vi "stc31-csv-to-data.vi"(10 "sensor-name":string, 11 "sensor-csv-input":string) -> (1 "STC31: Temp (degC)":dbl format="%.2f", 2 "STC31: CO2 (ppm)":dbl format="%.2f", 3 "STC31: data output":T1 {"CO2 (ppm)" format="%.2f"})   [LabVIEW 2021]
uses:
  STC31.ctl
  <vilib>/regexp/Match Regular Expression.xnode
panel:
  out "STC31: Temp":string
  out "STC31: CO2":string
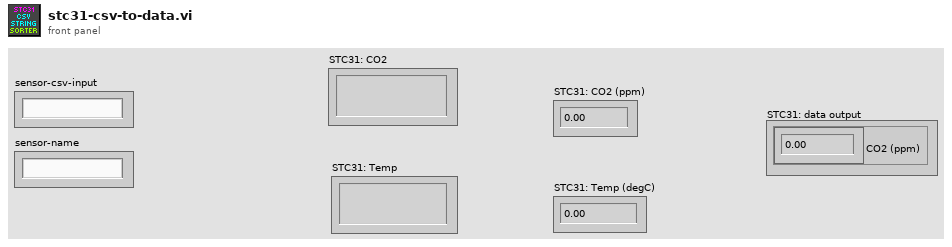
[diagram p1: front panel]
types:
  T1 = typedef "STC31.ctl" = cluster{"CO2 (ppm)":dbl}
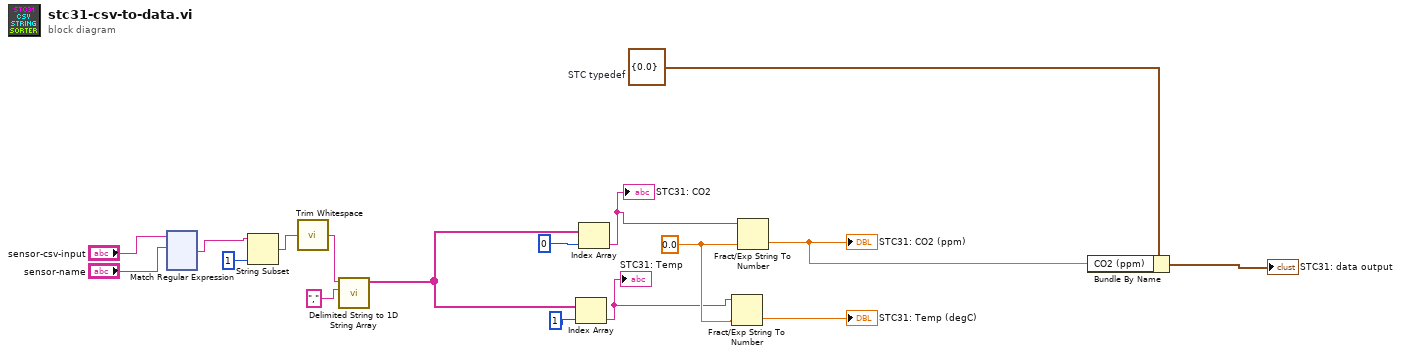
[diagram p0: block diagram]
diagram:
  w15 = T1 {"CO2 (ppm)"=0.0}  # STC typedef
  w17 = 0.0
  n1 = xnode "Match Regular Expression"("input string"="sensor-csv-input", "regular expression"="sensor-name") -> ("after match"=w1:string)  [unwired: 4 in, 4 out]
  n2 = String Subset(string=w1, offset (0)=1) -> (substring=w2:string)  [unwired: 1 in]
  n3 = call <vilib>:"Trim Whitespace.vi"("string"=w2) -> ("trimmed string"=w12:string)  [unwired: 1 in]
  n4 = call <vilib>:"Delimited String to 1D String Array.vi"("delimiter"=",", "delimited string"=w12) -> ("string array"=w6:string[])  [unwired: 9 in]
  n5 = Index Array(array=w6, index=1 ("y")) -> (element=w4:string)
  "STC31: Temp" <- w4
  n6 = Index Array "Index Array"(array=w6, index=0) -> (element=w5:string)
  "STC31: CO2" <- w5
  n7 = Fract/Exp String To Number(string=w4, default (0 dbl)=w17) -> (number=→"STC31: Temp (degC)":dbl)  [unwired: 2 in, 1 out]
  n8 = Fract/Exp String To Number(string=w5, default (0 dbl)=w17) -> (number=w14:dbl)  [unwired: 2 in, 1 out]
  "STC31: CO2 (ppm)" <- w14
  n9 = Bundle By Name(cluster=w15, "CO2 (ppm)"=w14) -> (→"STC31: data output":T1)
